vi "Actor Registry.vi"(6 "Actor Alias":string, 7 "Actor Core Name":string, 8 "Details":T3, 9 "Actor Enqueuer":refnum<class "Message Enqueuer.lvclass">, 10 "Actor ID":string, 11 "Action":T2) -> (0 "All Actors":T1[](array[typedef]), 1 "This Actor":T1, 3 "Found":bool, 4 "Actor Alias out":string, 5 "Event Registration Refnum":refnum<event-registration>)   [LabVIEW 2020, in "Actor Framework.lvlib"]
uses:
  Message Enqueuer/Message Enqueuer.lvclass
  Registration Mode.ctl
  This Actor.ctl
  Actor Framework.lvlib
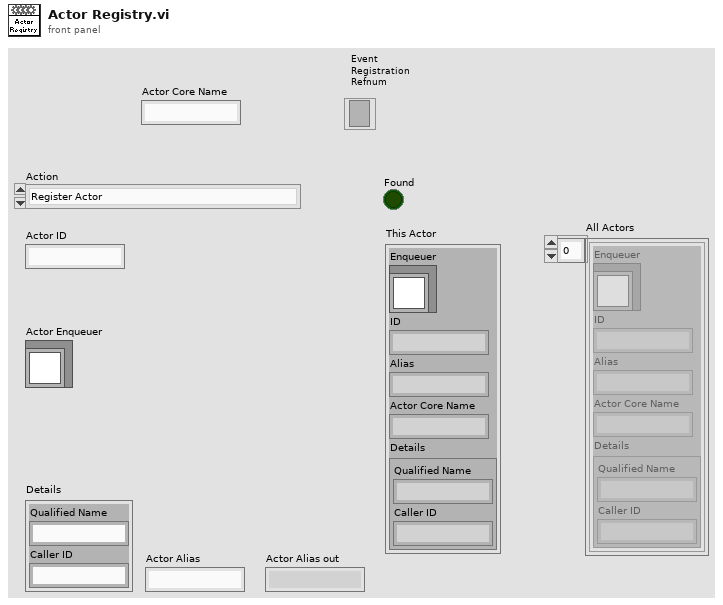
[diagram p1: front panel]
types:
  T1 = typedef "Actor Framework.lvlib/This Actor.ctl" = cluster{"Enqueuer":refnum<class "Message Enqueuer.lvclass">, "ID":string, "Alias":string, "Actor Core Name":string, "Details":cluster{"Qualified Name":string, "Caller ID":string}}
  T2 = typedef "Actor Framework.lvlib/Registration Mode.ctl" = enum16{"Register Actor", "Get ID", "Get Enqueuer", "Deregister Actor", "Get Update Event", "Get All Actors", "Set Actor Core Name"}
  T3 = cluster{"Qualified Name":string, "Caller ID":string}
  T4 = cluster{"Enqueuers":refnum<class "Message Enqueuer.lvclass">[], "IDs":string[], "Details":cluster{"Qualified Name":string, "Caller ID":string}[], "Aliases":string[], "Cores":string[], "Update Event":refnum<user-event>}
  T5 = cluster{"Qualified Name":string, "Caller ID":string}[]
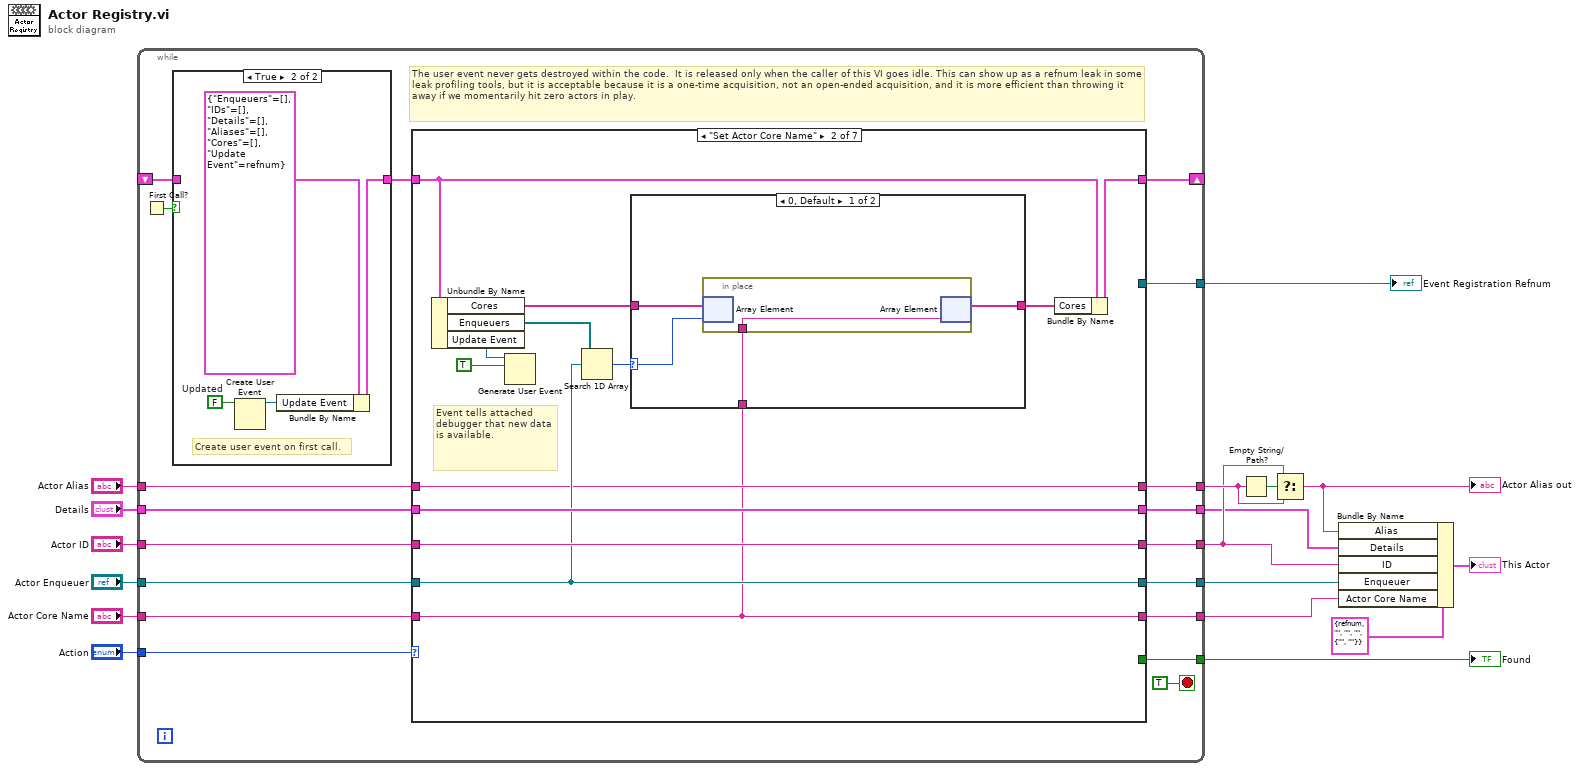
[diagram p0: block diagram]
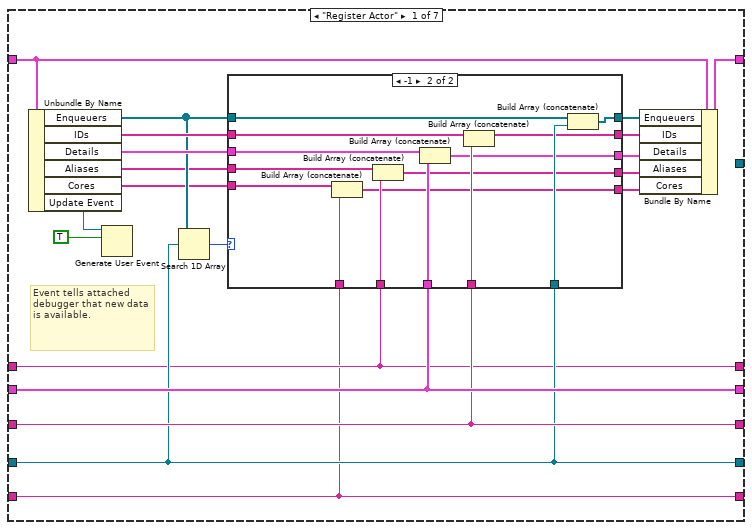
[diagram p3: hidden frame]
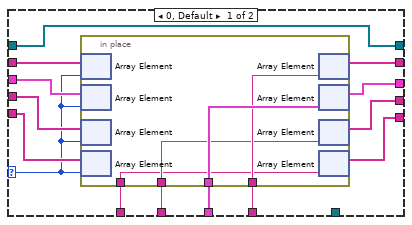
[diagram p4: hidden frame]
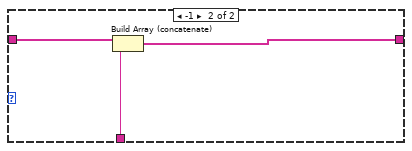
[diagram p5: hidden frame]
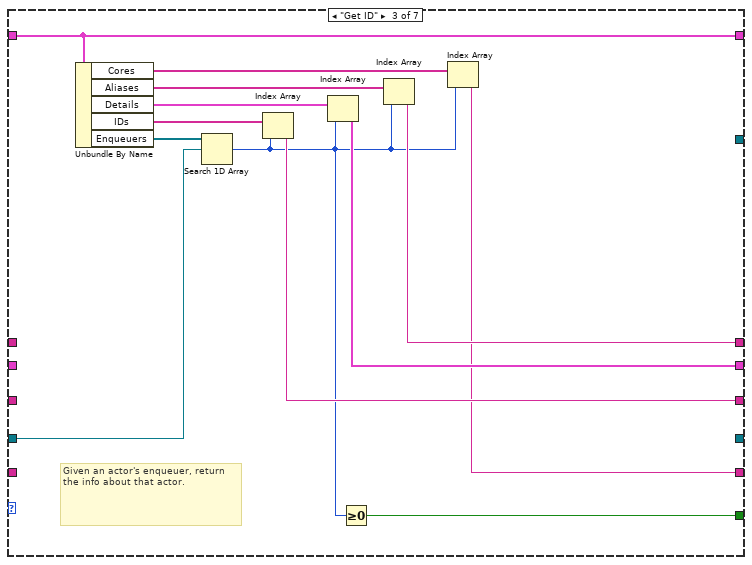
[diagram p6: hidden frame]
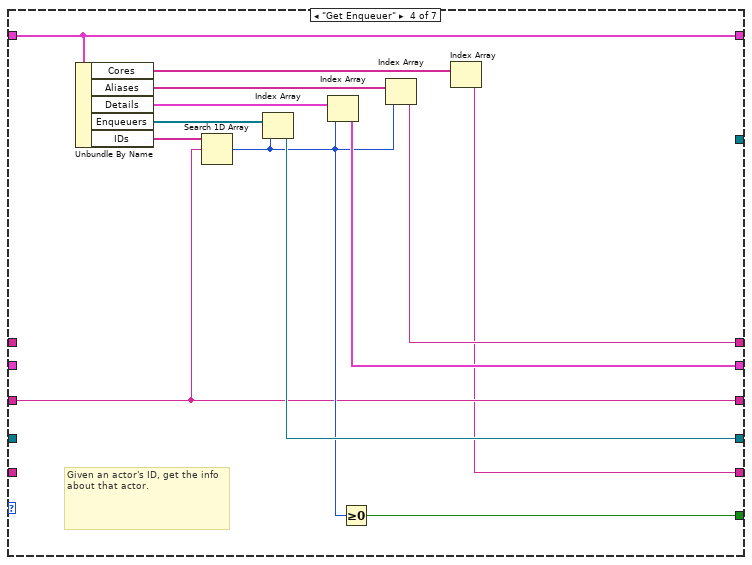
[diagram p7: hidden frame]
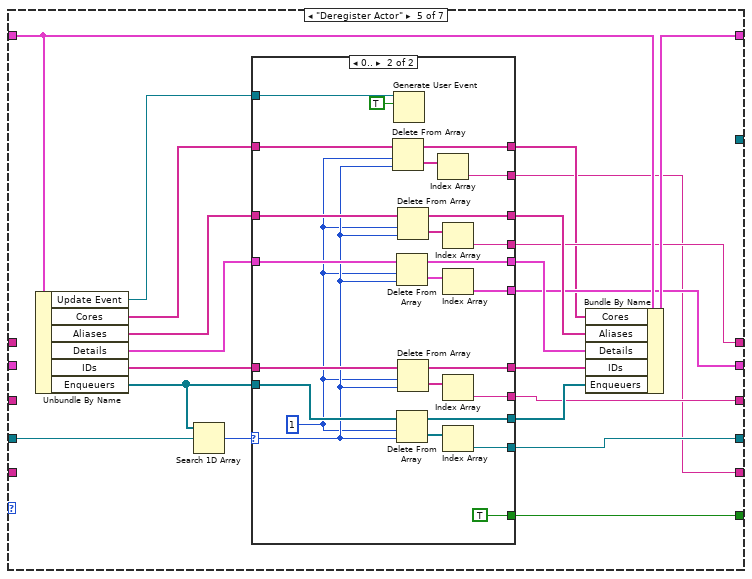
[diagram p8: hidden frame]
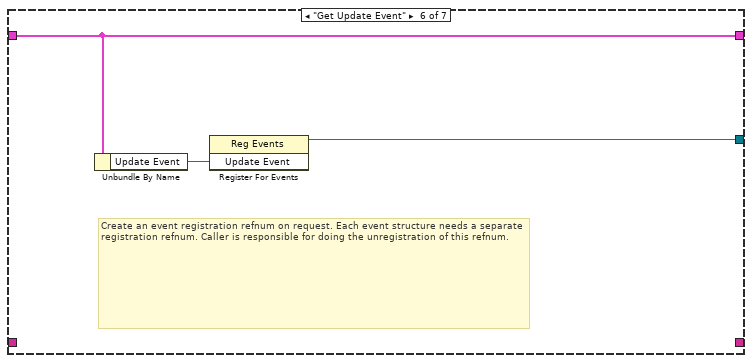
[diagram p10: hidden frame]
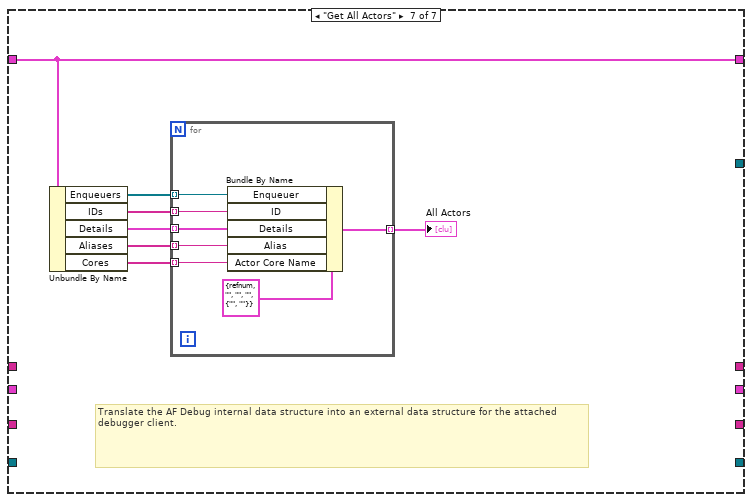
[diagram p11: hidden frame]
diagram:
  n1 = while {
    tunnel: "Action" -> [w35]
    shift-right: [w34] -> _
    shift-left: _ -> [w24]
    tunnel: "Actor ID" -> [w33]
    tunnel: "Actor Enqueuer" -> [w32]
    tunnel: "Details" -> [w31]
    tunnel: [w26] -> w8
    tunnel: [w29] -> w7
    tunnel: [w28] -> w13
    tunnel: [w27] -> w9
    tunnel: "Actor Alias" -> [w22]
    tunnel: [w21] -> w10
    tunnel: "Actor Core Name" -> [w20]
    tunnel: [w19] -> w3
    tunnel: [w18] -> w1
    stop <- TRUE stop-if-true
    # "The user event never gets destroyed within the code.  It is released only when the caller of this VI goes idle. This can show up as a refnum leak in some leak profiling tools, but it is acceptable because it is a one-time acquisition, not an open-ended acquisition, and it is more efficient than throwing it away if we momentarily hit zero actors in play."
    n2 = First Call?() -> (First Call?: T/F=w23:bool)
    n3 = case shown="True" w23 {
      tunnel: [w36 w39] -> w25
      tunnel: w24 -> [w36 _]
      frame False {
      }
      frame True {
        w40 = FALSE  # Updated
        # "Create user event on first call."
        n4 = Create User Event(user event datatype=w40) -> (user event=w38:refnum<user-event>)  [unwired: 1 in, 1 out]
        n5 = Bundle By Name(cluster=T4 {"Enqueuers"=[], "IDs"=[], "Details"=[], "Aliases"=[], "Cores"=[], "Update Event"=refnum}, "Update Event"=w38) -> (w39:T4)
      }
    }
    n6 = case shown="\"Set Actor Core Name\"" w35 {
      tunnel: w25 -> [w54 w105 w123 w137 w156 w194 w201]
      tunnel: [w60 w106 w123 w137 w151 w194 w201] -> w34
      tunnel: w33 -> [w48 w102 _ w131 _ _ _]
      tunnel: w32 -> [w47 w101 w126 _ w157 _ _]
      tunnel: w31 -> [w49 w103 _ _ _ _ _]
      tunnel: [w48 w102 w119 w131 w147 _ _] -> w26
      tunnel: [w49 w103 w121 w134 w145 _ _] -> w29
      tunnel: [_ _ w122 w136 w152 _ _] -> w28
      tunnel: [w47 w101 _ w135 w148 _ _] -> w27
      tunnel: w22 -> [w46 w100 _ _ _ _ _]
      tunnel: [w46 w100 w118 w130 w146 _ _] -> w21
      tunnel: w20 -> [w43 w97 _ _ _ _ _]
      tunnel: [w43 w97 w115 w128 w142 _ _] -> w19
      tunnel: [_ _ _ _ _ w192 _] -> w18
      frame "Register Actor" {
        # "Event tells attached debugger that new data is available."
        n7 = Unbundle By Name(w54) -> ("Enqueuers"=w53:refnum<class "Message Enqueuer.lvclass">[], "IDs"=w57:string[], "Details"=w56:T5, "Aliases"=w51:string[], "Cores"=w45:string[], "Update Event"=w42:refnum<user-event>)
        n8 = Generate User Event(user event=w42, event data cluster=TRUE ("event data")) -> ()  [unwired: 2 in, 2 out]
        n9 = Search 1D Array(1D array=w53, element=w47) -> (index of element=w52:i32)  [unwired: 1 in]
        n10 = case shown="-1" w52 {
          selector: w52 -> [w63 _]
          tunnel: w48 -> [w72 w93]
          tunnel: w47 -> [_ w92]
          tunnel: w49 -> [w73 w91]
          tunnel: w53 -> [w74 w90]
          tunnel: [w74 w89] -> w59
          tunnel: [w69 w88] -> w58
          tunnel: w57 -> [w71 w87]
          tunnel: w56 -> [w70 w86]
          tunnel: [w68 w85] -> w55
          tunnel: w51 -> [w67 w84]
          tunnel: [w66 w82] -> w50
          tunnel: w46 -> [w65 w83]
          tunnel: w45 -> [w64 w81]
          tunnel: [w62 w80] -> w44
          tunnel: w43 -> [w61 w79]
          frame 0, Default {
            n11 = in-place {
              in-place-border: w73 -> [w78]
              in-place-border: w72 -> [w77]
              in-place-border: w65 -> [w76]
              in-place-border: w61 -> [w75]
              n12 = in-place-array #1(w71, w63) -> ()  [unwired: 1 out]
              n13 = in-place-array #2(w70, w63) -> ()  [unwired: 1 out]
              n14 = in-place-array #3(w67, w63) -> ()  [unwired: 1 out]
              n15 = in-place-array #4(w64, w63) -> ()  [unwired: 1 out]
              n16 = in-place-array #1(w77) -> (w69:string[])  [unwired: 1 out]
              n17 = in-place-array #2(w78) -> (w68:T5)  [unwired: 1 out]
              n18 = in-place-array #3(w76) -> (w66:string[])  [unwired: 1 out]
              n19 = in-place-array #4(w75) -> (w62:string[])  [unwired: 1 out]
            }
          }
          frame -1 {
            n20 = Build Array (concatenate)(w81, w79) -> (w80:string[])
            n21 = Build Array (concatenate)(w84, w83) -> (w82:string[])
            n22 = Build Array (concatenate)(w86, w91) -> (w85:T5)
            n23 = Build Array (concatenate)(w87, w93) -> (w88:string[])
            n24 = Build Array (concatenate)(w90, w92) -> (w89:refnum<class "Message Enqueuer.lvclass">[])
          }
        }
        n25 = Bundle By Name(cluster=w54, "Enqueuers"=w59, "IDs"=w58, "Details"=w55, "Aliases"=w50, "Cores"=w44) -> (w60:T4)
      }
      frame "Set Actor Core Name" {
        # "Event tells attached debugger that new data is available."
        n26 = Unbundle By Name(w105) -> ("Cores"=w99:string[], "Enqueuers"=w94:refnum<class "Message Enqueuer.lvclass">[], "Update Event"=w96:refnum<user-event>)
        n27 = Generate User Event(user event=w96, event data cluster=TRUE ("event data")) -> ()  [unwired: 2 in, 2 out]
        n28 = Search 1D Array(1D array=w94, element=w101) -> (index of element=w104:i32)  [unwired: 1 in]
        n29 = case shown="0, Default" w104 {
          selector: w104 -> [w109 _]
          tunnel: w99 -> [w110 w114]
          tunnel: [w108 w113] -> w98
          tunnel: w97 -> [w107 w112]
          frame 0, Default {
            n30 = in-place {
              in-place-border: w107 -> [w111]
              n31 = in-place-array #5(w110, w109) -> ()  [unwired: 1 out]
              n32 = in-place-array #5(w111) -> (w108:string[])  [unwired: 1 out]
            }
          }
          frame -1 {
            n33 = Build Array (concatenate)(w114, w112) -> (w113:string[])
          }
        }
        n34 = Bundle By Name(cluster=w105, "Cores"=w98) -> (w106:T4)
      }
      frame "Get ID" {
        # "Given an actor's enqueuer, return the info about that actor."
        n35 = Unbundle By Name(w123) -> ("Cores"=w117:string[], "Aliases"=w120:string[], "Details"=w125:T5, "IDs"=w124:string[], "Enqueuers"=w127:refnum<class "Message Enqueuer.lvclass">[])
        n36 = Search 1D Array(1D array=w127, element=w126) -> (index of element=w116:i32)  [unwired: 1 in]
        n37 = Index Array(array=w124, index=w116) -> (element=w119:string)
        n38 = Index Array(array=w125, index=w116) -> (element=w121:T3)
        n39 = Greater Or Equal To 0?(x=w116) -> (x >= 0?=w122:bool)
        n40 = Index Array(array=w120, index=w116) -> (element=w118:string)
        n41 = Index Array(array=w117, index=w116) -> (element=w115:string)
      }
      frame "Get Enqueuer" {
        # "Given an actor's ID, get the info about that actor."
        n42 = Unbundle By Name(w137) -> ("Cores"=w129:string[], "Aliases"=w133:string[], "Details"=w139:T5, "Enqueuers"=w138:refnum<class "Message Enqueuer.lvclass">[], "IDs"=w140:string[])
        n43 = Search 1D Array(1D array=w140, element=w131) -> (index of element=w132:i32)  [unwired: 1 in]
        n44 = Index Array(array=w138, index=w132) -> (element=w135:refnum<class "Message Enqueuer.lvclass">)
        n45 = Index Array(array=w139, index=w132) -> (element=w134:T3)
        n46 = Greater Or Equal To 0?(x=w132) -> (x >= 0?=w136:bool)
        n47 = Index Array(array=w133, index=w132) -> (element=w130:string)
        n48 = Index Array(array=w129) -> (element=w128:string)  [unwired: 1 in]
      }
      frame "Deregister Actor" {
        n49 = Unbundle By Name(w156) -> ("Update Event"=w141:refnum<user-event>, "Cores"=w144:string[], "Aliases"=w150:string[], "Details"=w159:T5, "IDs"=w158:string[], "Enqueuers"=w160:refnum<class "Message Enqueuer.lvclass">[])
        n50 = Search 1D Array(1D array=w160, element=w157) -> (index of element=w161:i32)  [unwired: 1 in]
        n51 = case shown="0.." w161 {
          selector: w161 -> [_ w170]
          tunnel: [w165 w191] -> w154
          tunnel: w160 -> [w166 w190]
          tunnel: [w166 w189] -> w155
          tunnel: w158 -> [w165 w188]
          tunnel: [_ TRUE] -> w152
          tunnel: w159 -> [w164 w186]
          tunnel: [w164 w185] -> w153
          tunnel: w150 -> [w163 w184]
          tunnel: [w163 w183] -> w149
          tunnel: [_ w178] -> w148
          tunnel: [_ w177] -> w147
          tunnel: [_ w176] -> w146
          tunnel: [_ w175] -> w145
          tunnel: w144 -> [w162 w173]
          tunnel: [w162 w172] -> w143
          tunnel: [_ w171] -> w142
          tunnel: w141 -> [_ w167]
          frame ..-1 {
          }
          frame 0.. {
            w169 = 1 ("length")
            n52 = Delete From Array(array=w173, length=w169, index=w170) -> (deleted portion=w174:string[], array with subset deleted=w172:string[])
            n53 = Generate User Event(user event=w167, event data cluster=TRUE ("event data")) -> ()  [unwired: 2 in, 2 out]
            n54 = Delete From Array(array=w186, length=w169, index=w170) -> (deleted portion=w181:T5, array with subset deleted=w185:T5)
            n55 = Delete From Array(array=w190, length=w169, index=w170) -> (deleted portion=w179:refnum<class "Message Enqueuer.lvclass">[], array with subset deleted=w189:refnum<class "Message Enqueuer.lvclass">[])
            n56 = Delete From Array(array=w184, length=w169, index=w170) -> (deleted portion=w182:string[], array with subset deleted=w183:string[])
            n57 = Delete From Array(array=w188, length=w169, index=w170) -> (deleted portion=w180:string[], array with subset deleted=w191:string[])
            n58 = Index Array(array=w174) -> (element=w171:string)  [unwired: 1 in]
            n59 = Index Array(array=w182) -> (element=w176:string)  [unwired: 1 in]
            n60 = Index Array(array=w181) -> (element=w175:T3)  [unwired: 1 in]
            n61 = Index Array(array=w180) -> (element=w177:string)  [unwired: 1 in]
            n62 = Index Array(array=w179) -> (element=w178:refnum<class "Message Enqueuer.lvclass">)  [unwired: 1 in]
          }
        }
        n63 = Bundle By Name(cluster=w156, "Cores"=w143, "Aliases"=w149, "Details"=w153, "IDs"=w154, "Enqueuers"=w155) -> (w151:T4)
      }
      frame "Get Update Event" {
        # "Create an event registration refnum on request. Each event structure needs a separate registration refnum. Caller is responsible for doing the unregistration of this refnum."
        n64 = Unbundle By Name(w194) -> ("Update Event"=w193:refnum<user-event>)
        n65 = register-events(w193) -> (reference out=w192:refnum<event-registration>)  [unwired: 2 in, 1 out]
      }
      frame "Get All Actors" {
        # "Translate the AF Debug internal data structure into an external data structure for the attached debugger client."
        n66 = Unbundle By Name(w201) -> ("Enqueuers"=w200:refnum<class "Message Enqueuer.lvclass">[], "IDs"=w199:string[], "Details"=w198:T5, "Aliases"=w197:string[], "Cores"=w196:string[])
        n67 = for {
          tunnel: w200 -> [w207] mode=indexing
          tunnel: w199 -> [w206] mode=indexing
          tunnel: w198 -> [w205] mode=indexing
          tunnel: w197 -> [w204] mode=indexing
          tunnel: w196 -> [w203] mode=indexing
          tunnel: [w202] -> w195 mode=indexing
          n68 = Bundle By Name(cluster=T1 {"Enqueuer"=refnum, "ID"="", "Alias"="", "Actor Core Name"="", "Details"={"Qualified Name"="", "Caller ID"=""}} ("This Actor"), "Enqueuer"=w207, "ID"=w206, "Details"=w205, "Alias"=w204, "Actor Core Name"=w203) -> (w202:T1)
        }
        "All Actors" <- w195
      }
    }
  }
  "Found" <- w13
  "Event Registration Refnum" <- w1
  n69 = Empty String/Path?(string/path=w10) -> (empty?=w11:bool)
  n70 = Select(t=w8, s=w11, f=w10) -> (s? t:f=w6:string)
  "Actor Alias out" <- w6
  n71 = Bundle By Name(cluster=T1 {"Enqueuer"=refnum, "ID"="", "Alias"="", "Actor Core Name"="", "Details"={"Qualified Name"="", "Caller ID"=""}} ("This Actor"), "Alias"=w6, "Details"=w7, "ID"=w8, "Enqueuer"=w9, "Actor Core Name"=w3) -> (→"This Actor":T1)
